vi "touchTester.vi"(0 "Input":T1) -> (1 "String":string, 2 "NXT/EV3":T1, 3 "RGB Color":cluster{"Red":u8, "Green":u8, "Blue":u8})   [LabVIEW 2016]
uses:
  <vilib>/NXT/Subs/LVHSConnector.ctl
  <vilib>/NXT/LegoClasses/BrickReference/BrickReference.lvclass
  <vilib>/NXT/Block Support/NXT_InputPort.ctl
  <vilib>/NXT/Block Support/NXT_OutputPort.ctl
  <vilib>/NXT/Dual Mode Library/Waits/Wait_Num.vi
  <vilib>/NXT/NXTIO Xnodes/NXTIONodeSubVIs/NXTMotorRunDistance.vi
  <vilib>/NXT/Dual Mode Library/Sensors/Touch_Pressed.vi
  <vilib>/NXT/Dual Mode Library/Sensors/EV3_Color_RGB.vi
  <vilib>/NXT/NXTIO Xnodes/AddressXNode/NXTIOAddress.xnode
  <vilib>/NXT/NXTIO Xnodes/NXTIOXNode/NXTIO.xnode
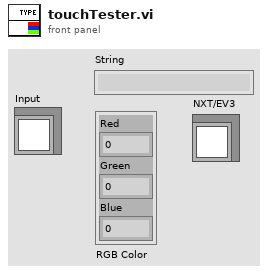
[diagram p1: front panel]
types:
  T1 = typedef "LVHSConnector.ctl" = refnum<class "BrickReference.lvclass">
  T2 = typedef "NXT_InputPort.ctl" = u32
  T3 = typedef "NXT_OutputPort.ctl" = u8
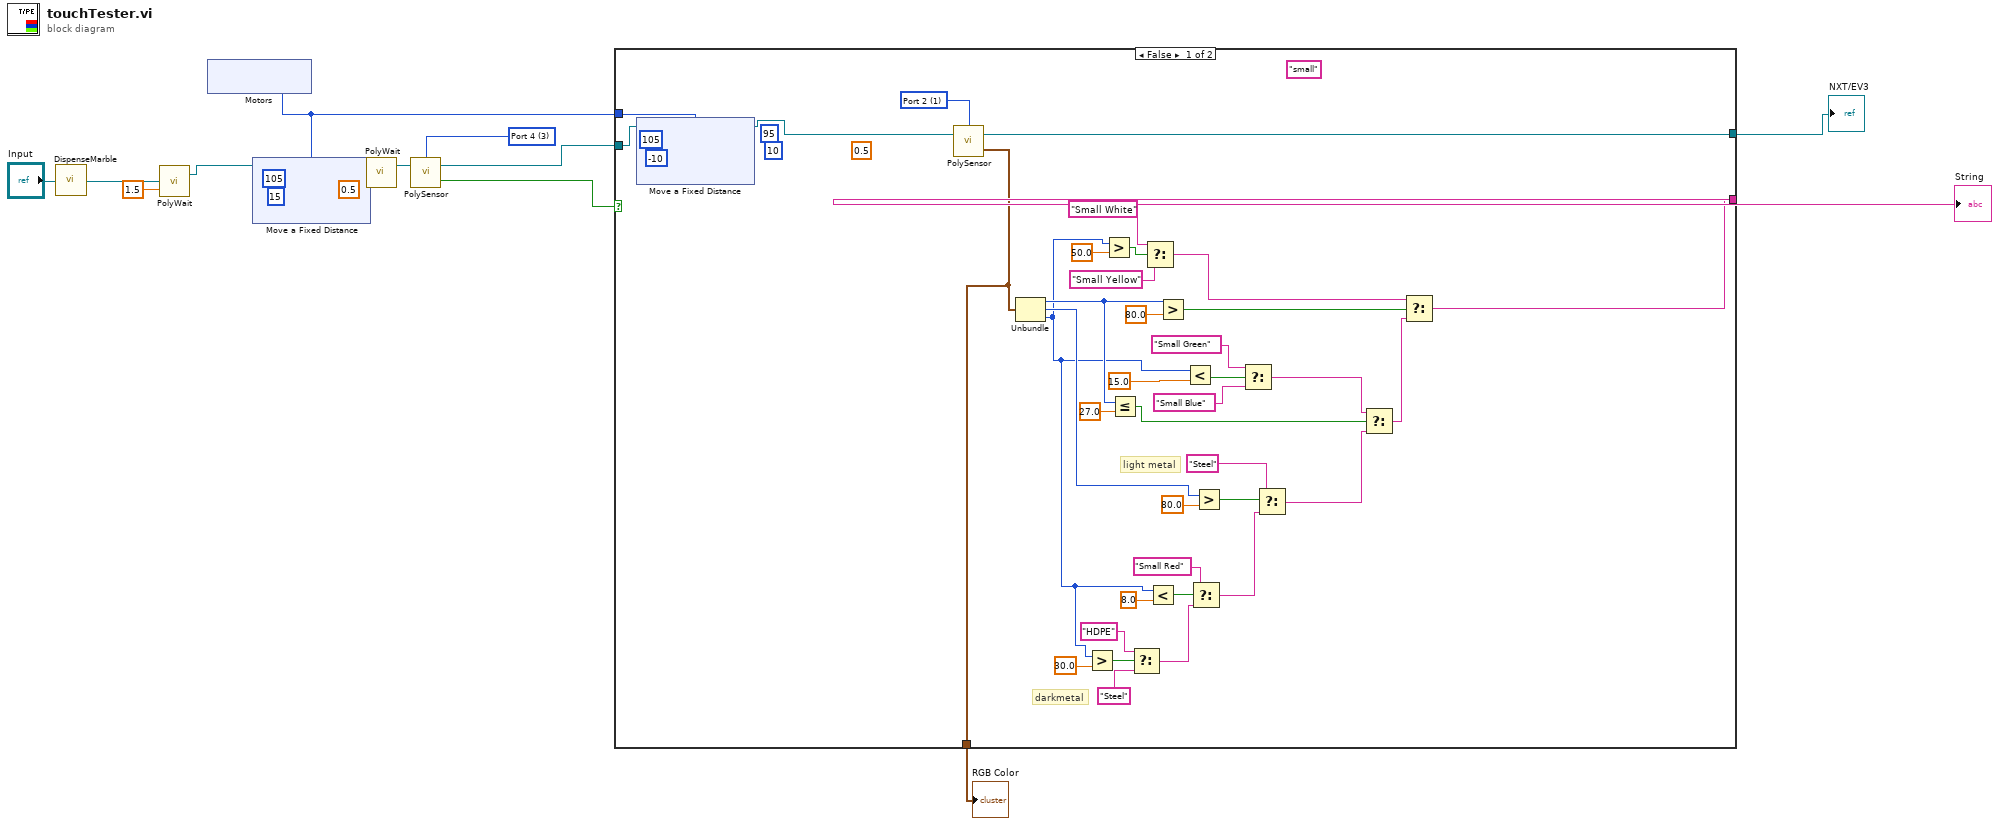
[diagram p0: block diagram]
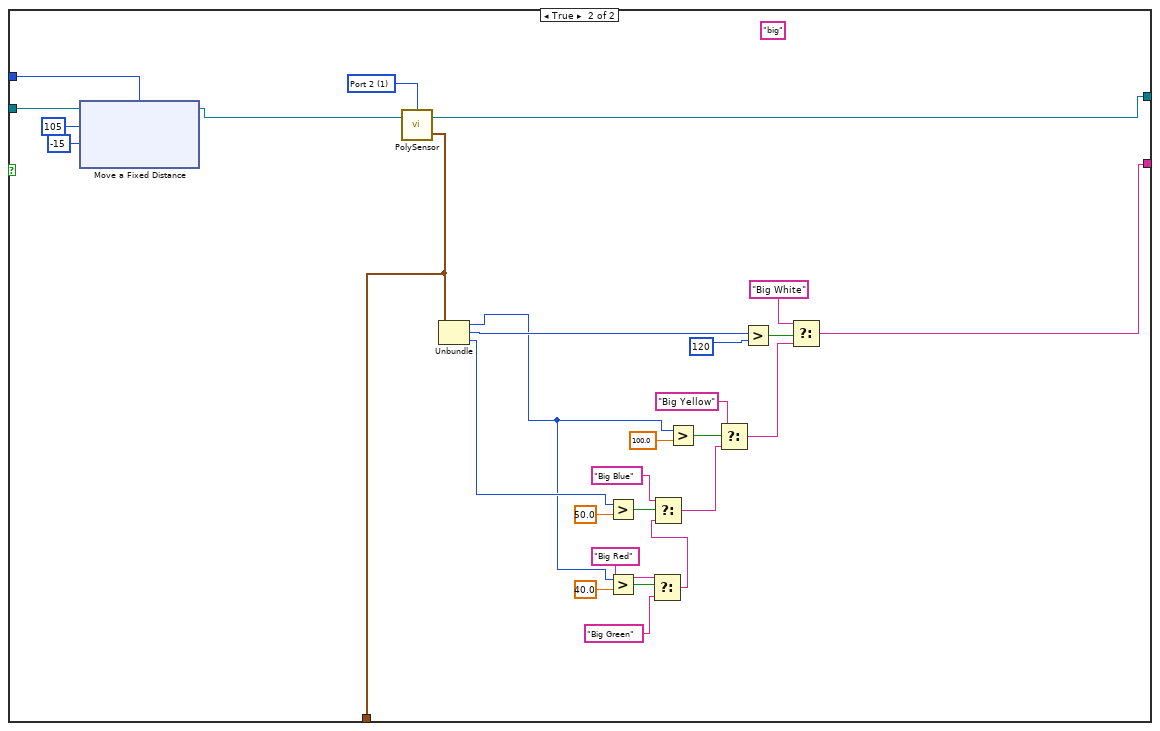
[diagram p2: hidden frame]
diagram:
  w16 = T2 3 items=["Port 1", "Port 2", "Port 3", "Port 4"] ("Port (Port 1)")
  n1 = call "DispenseMarble.vi"("Input"="Input") -> ("Output"=w4:T1)
  n2 = call-poly <vilib>:"PolyWait.vi"("Time (1 sec)"=sgl 1.5, "NXT/EV3"=w4) -> ("NXT/EV3"=w3:T1)  [unwired: 2 in]
  n3 = xnode "Motors"() -> ("Motor"=w8:T3)
  n4 = xnode "Move a Fixed Distance"("Speed 1"=i8 15, "Distance 1"=105, "Motors"=w8, "NXT/EV3"=w3) -> ("NXT/EV3"=w14:T1)  [unwired: 1 in]
  n5 = call-poly <vilib>:"PolyWait.vi"("Time (1 sec)"=sgl 0.5, "NXT/EV3"=w14) -> ("NXT/EV3"=w13:T1)  [unwired: 2 in]
  n6 = call-poly <vilib>:"PolySensor.vi"("NXT/EV3"=w13, "Port (Port 1)"=w16) -> ("Yes / No"=w12:bool, "NXT/EV3"=w9:T1)  [unwired: 1 in]
  n7 = case shown="False" w12 {
    tunnel: [w19 w70] -> w11
    tunnel: w9 -> [w54 w93]
    tunnel: w8 -> [w53 w92]
    tunnel: [w51 w90] -> w6
    tunnel: [w17 w68] -> w1
    frame False {
      w18 = T2 1 items=["Port 1", "Port 2", "Port 3", "Port 4"] ("Port (Port 1)")
      (unwired) sgl 0.5 ("Time (1 sec)")
      (unwired) 95 ("Distance 1")
      (unwired) i8 10 ("Speed 1")
      (unwired) "small" ("String")
      # "darkmetal"
      # "light metal"
      n8 = xnode "Move a Fixed Distance"("Speed 1"=i8 -10, "Distance 1"=105, "Motors"=w53, "NXT/EV3"=w54) -> ("NXT/EV3"=w52:T1)  [unwired: 1 in]
      n9 = call-poly <vilib>:"PolySensor.vi"("NXT/EV3"=w52, "Port (Port 1)"=w18) -> ("RGB Color"=w51:cluster{"Red":u8, "Green":u8, "Blue":u8}, "NXT/EV3"=w17:T1)  [unwired: 1 in]
      n10 = Unbundle(w51) -> ("Red"=w42:u8, "Green"=w32:u8, "Blue"=w21:u8)
      n11 = Greater?(x=w21, y=30.0) -> (0:w24:bool)
      n12 = Greater?(x=w21, y=50.0) -> (0:w46:bool)
      n13 = Less Or Equal?(x=w42, y=27.0) -> (x <= y?=w41:bool)
      n14 = Select(t="HDPE", s=w24, f="Steel") -> (s? t:f=w25:string)
      n15 = Select(t="Small White", s=w46, f="Small Yellow") -> (s? t:f=w48:string)
      n16 = Less?(x=w21, y=8.0) -> (x < y?=w28:bool)
      n17 = Greater?(x=w42, y=80.0) -> (0:w50:bool)
      n18 = Less?(x=w21, y=15.0) -> (x < y?=w40:bool)
      n19 = Select(t="Small Red", s=w28, f=w25) -> (s? t:f=w29:string)
      n20 = Greater?(x=w32, y=80.0) -> (0:w33:bool)
      n21 = Select(t="Small Green", s=w40, f="Small Blue") -> (s? t:f=w38:string)
      n22 = Select(t="Steel", s=w33, f=w29) -> (s? t:f=w35:string)
      n23 = Select(t=w38, s=w41, f=w35) -> (s? t:f=w30:string)
      n24 = Select(t=w48, s=w50, f=w30) -> (s? t:f=w19:string)
    }
    frame True {
      w69 = T2 1 items=["Port 1", "Port 2", "Port 3", "Port 4"] ("Port (Port 1)")
      (unwired) "big"
      n25 = xnode "Move a Fixed Distance"("Speed 1"=i8 -15, "Distance 1"=105, "Motors"=w92, "NXT/EV3"=w93) -> ("NXT/EV3"=w91:T1)  [unwired: 1 in]
      n26 = call-poly <vilib>:"PolySensor.vi"("NXT/EV3"=w91, "Port (Port 1)"=w69) -> ("RGB Color"=w90:cluster{"Red":u8, "Green":u8, "Blue":u8}, "NXT/EV3"=w68:T1)  [unwired: 1 in]
      n27 = Unbundle(w90) -> ("Red"=w75:u8, "Green"=w87:u8, "Blue"=w80:u8)
      n28 = Greater?(x=w80, y=50.0) -> (0:w79:bool)
      n29 = Greater?(x=w75, y=40.0) -> (0:w74:bool)
      n30 = Select(t="Big Red", s=w74, f="Big Green") -> (s? t:f=w71:string)
      n31 = Select(t="Big Blue", s=w79, f=w71) -> (s? t:f=w77:string)
      n32 = Greater?(x=w75, y=100.0) -> (0:w83:bool)
      n33 = Select(t="Big Yellow", s=w83, f=w77) -> (s? t:f=w85:string)
      n34 = Greater?(x=w87, y=120) -> (0:w89:bool)
      n35 = Select(t="Big White", s=w89, f=w85) -> (s? t:f=w70:string)
    }
  }
  "String" <- w11
  "RGB Color" <- w6
  "NXT/EV3" <- w1
